vi "reprTextual.vi"(8 "error in (no error)":errorcluster, 11 "PassBuoys in":refnum<class "PassBuoys.lvclass">) -> (0 "error out":errorcluster, 2 "Description":string, 3 "PassBuoys out":refnum<class "PassBuoys.lvclass">)   [LabVIEW 2011, in "PassBuoys.lvclass"]
uses:
  PassBuoys.lvclass
  PassBuoys.lvclass/PassBuoys.ctl
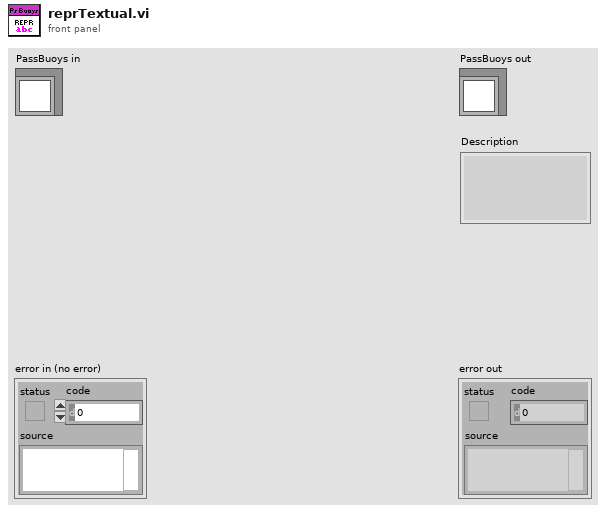
[diagram p1: front panel]
types:
  T1 = typedef "UTM Location.ctl" = cluster{"UTM Zone":dbl, "Hemisphere":enum16{"North", "South"}, "East":dbl, "North":dbl}
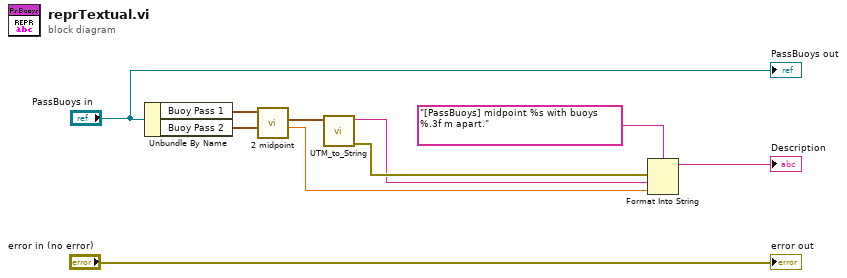
[diagram p0: block diagram]
diagram:
  n1 = Unbundle By Name("PassBuoys in") -> ("Buoy Pass 1"=w5:T1, "Buoy Pass 2"=w4:T1)
  n2 = call "2 midpoint.vi"("UTM 2"=w4, "UTM 1"=w5) -> ("Distance"=w2:dbl, "Midpoint"=w3:T1)  [unwired: 8 in]
  n3 = call "UTM_to_String.vi"("UTM Location"=w3) -> ("error out"=w8:errorcluster, "UTM String"=w7:string)  [unwired: 9 in]
  n4 = Format Into String(format string="[PassBuoys] midpoint %s with buoys %.3f m apart.", error in=w8, w7, w2) -> (resulting string=→"Description":string)  [unwired: 1 in, 1 out]
  "error out" <- "error in (no error)"
  "PassBuoys out" <- "PassBuoys in"
